vi "XBOX_Joystick_Name.vi"(9 "POVs":i16[](array[numeric]), 10 "Buttons":bool[](array[boolean]), 11 "Axes":dbl[](array[numeric])) -> (2 "Named Axes":T1, 3 "Named Buttons":T2)   [LabVIEW 2017, in "ArgosLib.lvlib"]
uses:
  ArgosLib.lvlib
  TypeDefs/XBoxButtons_Type.ctl
  TypeDefs/XBoxAxes_Type.ctl
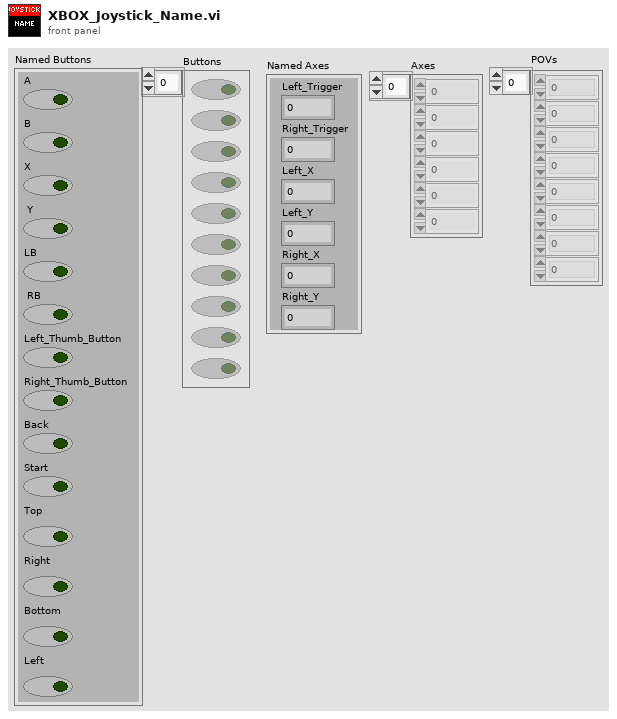
[diagram p1: front panel]
types:
  T1 = typedef "ArgosLib.lvlib/XBoxAxes_Type.ctl" = cluster{"Left_Trigger":dbl, "Right_Trigger ":dbl, "Left_X":dbl, "Left_Y":dbl, "Right_X":dbl, "Right_Y":dbl}
  T2 = typedef "ArgosLib.lvlib/XBoxButtons_Type.ctl" = cluster{"A":bool, "B":bool, "X":bool, " Y":bool, "LB":bool, " RB":bool, "Left_Thumb_Button":bool, "Right_Thumb_Button":bool, "Back":bool, "Start":bool, "Top":bool, "Right":bool, "Bottom":bool, "Left":bool}
  T3 = cluster{"Axes[0]":dbl, "Axes[1]":dbl, "Axes[2]":dbl, "Axes[3]":dbl, "Axes[4]":dbl, "Axes[5]":dbl}
  T4 = cluster{"Buttons[0]":bool, "Buttons[1]":bool, "Buttons[2]":bool, "Buttons[3]":bool, "Buttons[4]":bool, "Buttons[5]":bool, "Buttons[6]":bool, "Buttons[7]":bool, "Buttons[8]":bool, "Buttons[9]":bool}
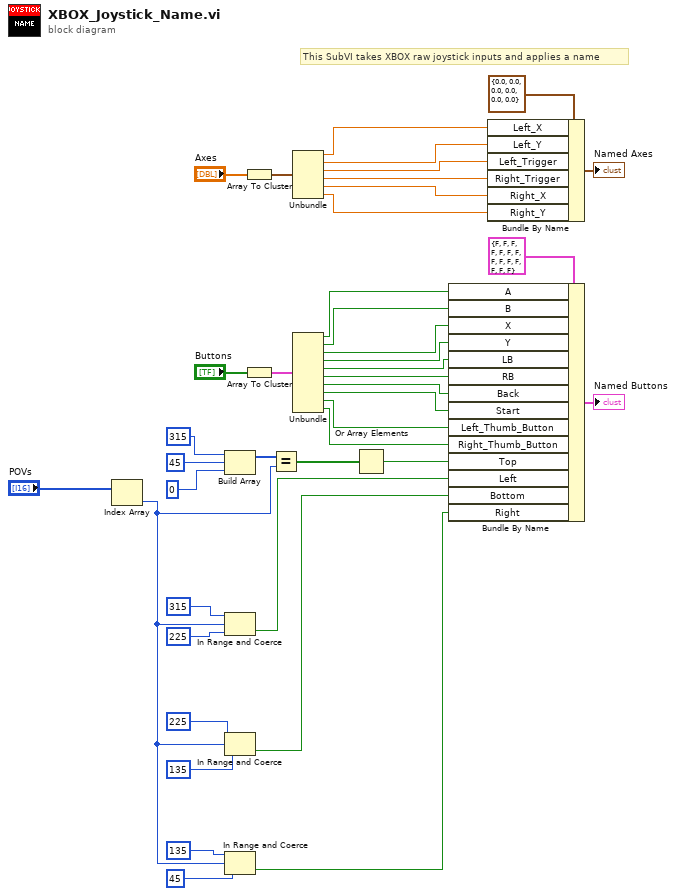
[diagram p0: block diagram]
diagram:
  # "This SubVI takes XBOX raw joystick inputs and applies a name"
  n1 = Index Array(array="POVs") -> (element=w2:i16)  [unwired: 1 in]
  n2 = Build Array(i16 315 ("upper limit"), i16 45 ("element"), i16 0 ("element")) -> (w3:i16[])
  n3 = In Range and Coerce(upper limit=i16 315, x=w2, lower limit=i16 225) -> (In Range?=w10:bool)  [unwired: 1 out]
  n4 = In Range and Coerce(upper limit=i16 225, x=w2, lower limit=i16 135) -> (In Range?=w9:bool)  [unwired: 1 out]
  n5 = In Range and Coerce(upper limit=i16 135, x=w2, lower limit=i16 45) -> (In Range?=w8:bool)  [unwired: 1 out]
  n6 = Array To Cluster(array="Axes") -> (cluster=w24:T3)
  n7 = Array To Cluster(array="Buttons") -> (cluster=w21:T4)
  n8 = Equal?(x=w3, y=w2) -> (x = y?=w4:bool[])
  n9 = Unbundle(w24) -> ("Axes[0]"=w36:dbl, "Axes[1]"=w37:dbl, "Axes[2]"=w38:dbl, "Axes[3]"=w39:dbl, "Axes[4]"=w40:dbl, "Axes[5]"=w41:dbl)
  n10 = Unbundle(w21) -> ("Buttons[0]"=w26:bool, "Buttons[1]"=w27:bool, "Buttons[2]"=w28:bool, "Buttons[3]"=w29:bool, "Buttons[4]"=w30:bool, "Buttons[5]"=w31:bool, "Buttons[6]"=w32:bool, "Buttons[7]"=w33:bool, "Buttons[8]"=w34:bool, "Buttons[9]"=w20:bool)
  n11 = Or Array Elements(Boolean array=w4) -> (logical OR=w1:bool)
  n12 = Bundle By Name(cluster=T2 {"A"=FALSE, "B"=FALSE, "X"=FALSE, " Y"=FALSE, "LB"=FALSE, " RB"=FALSE, "Left_Thumb_Button"=FALSE, "Right_Thumb_Button"=FALSE, "Back"=FALSE, "Start"=FALSE, "Top"=FALSE, "Right"=FALSE, "Bottom"=FALSE, "Left"=FALSE}, "A"=w26, "B"=w27, "X"=w28, "Y"=w29, "LB"=w30, "RB"=w31, "Back"=w32, "Start"=w33, "Left_Thumb_Button"=w34, "Right_Thumb_Button"=w20, "Top"=w1, "Left"=w10, "Bottom"=w9, "Right"=w8) -> (→"Named Buttons":T2)
  n13 = Bundle By Name(cluster=T1 {"Left_Trigger"=0.0, "Right_Trigger "=0.0, "Left_X"=0.0, "Left_Y"=0.0, "Right_X"=0.0, "Right_Y"=0.0}, "Left_X"=w36, "Left_Y"=w37, "Left_Trigger"=w38, "Right_Trigger"=w39, "Right_X"=w40, "Right_Y"=w41) -> (→"Named Axes":T1)
